vi "G#Object_Clone.vi"(0 "reference in":refnum<class "G#Object.lvclass">, 1 "new object name":string, 4 "no registration? (F)":bool, 5 "error in (no error)":errorcluster, 7 "user counter (T)?":bool=TRUE) -> (14 "reference out":refnum<class "G#Object.lvclass">, 16 "new object reference out":refnum<class "G#Object.lvclass">, 19 "error out":errorcluster)   [LabVIEW 2020, in "G#Object.lvclass"]
doc: "Clones the object specified by reference in and creates a new object with the identical state."
uses:
  G#Object.lvclass
  G#Object_State.ctl
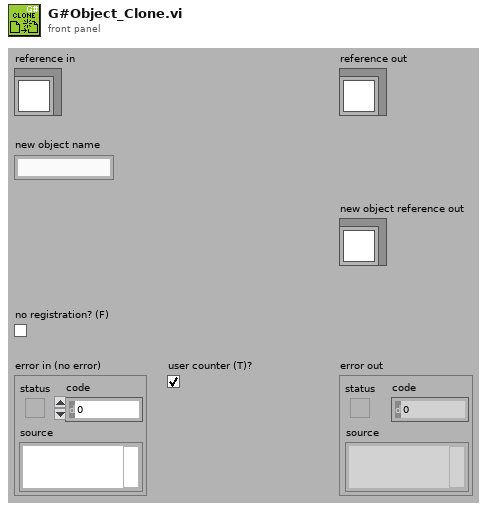
[diagram p1: front panel]
types:
  T1 = typedef "G#Object.lvclass/G#Object_State.ctl" = enum16{"Clear", "Create", "Delete", "Get class attributes", "Class hierarchy", "Get attribute value", "Set attribute value"}
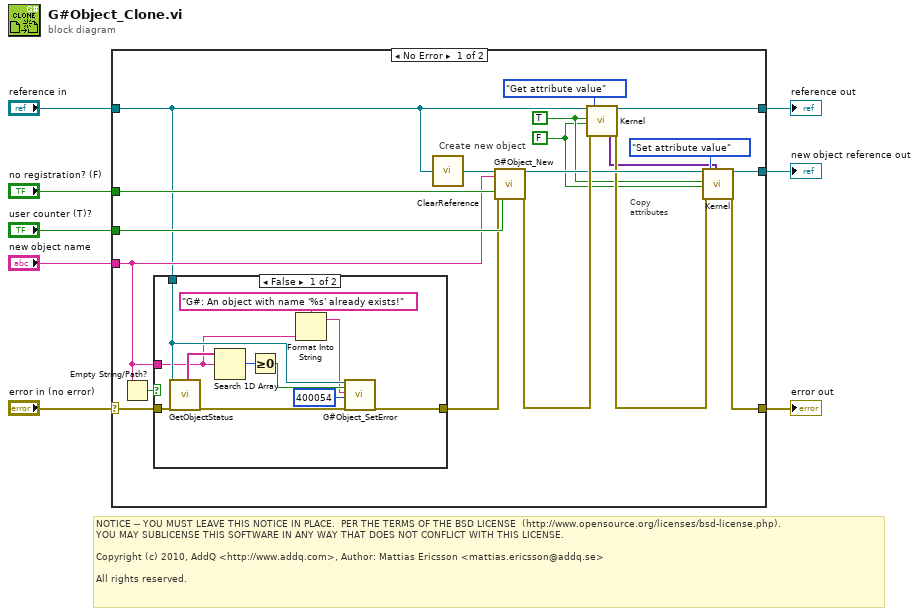
[diagram p0: block diagram]
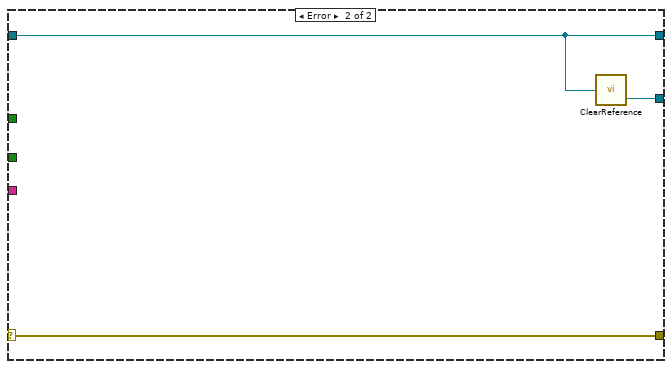
[diagram p3: hidden frame]
diagram:
  # "NOTICE -- YOU MUST LEAVE THIS NOTICE IN PLACE.  PER THE TERMS OF THE BSD LICENSE  (http://www.opensource.org/licenses/bsd-license.php).\nYOU MAY SUBLICENSE THIS SOFTWARE IN ANY WAY THAT DOES NOT CONFLICT WITH THIS LICENSE.\n\nCopyright (c) 2010, AddQ <http://www.addq.com>, Author: Mattias Ericsson <mattias.ericsson@addq.se>\n\nAll rights reserved."
  n1 = case shown="No Error" "error in (no error)" {
    selector: "error in (no error)" -> [w24 w42]
    tunnel: [w15 w42] -> w7
    tunnel: [w14 w40] -> w5
    tunnel: "reference in" -> [w20 w40]
    tunnel: "new object name" -> [w21 _]
    tunnel: "no registration? (F)" -> [w27 _]
    tunnel: "user counter (T)?" -> [w26 _]
    tunnel: [w18 w41] -> w1
    frame No Error {
      w9 = FALSE ("option 2")
      w10 = TRUE ("option 1")
      # "Copy\nattributes"
      # "Create new object"
      n2 = Empty String/Path?(string/path=w21) -> (empty?=w22:bool)
      n3 = case shown="False" w22 {
        tunnel: w24 -> [w38 w39]
        tunnel: [w35 w39] -> w23
        tunnel: w20 -> [w34 _]
        tunnel: w21 -> [w28 _]
        frame False {
          n4 = call-dynamic "GetObjectStatus.vi"("reference in"=w34, "error in (no error)"=w38) -> ("all object names"=w37:string[], "error out"=w36:errorcluster)  [unwired: 6 in, 10 out]
          n5 = Search 1D Array(1D array=w37, element=w28) -> (index of element=w33:i32)  [unwired: 1 in]
          n6 = Greater Or Equal To 0?(x=w33) -> (x >= 0?=w32:bool)
          n7 = Format Into String(format string="G#: An object with name '%s' already exists!", w28) -> (resulting string=w29:string)  [unwired: 2 in, 1 out]
          n8 = call "G#Object_SetError.vi"("reference in"=w34, "error (F)"=w32, "source"=w29, "code"=400054, "error in (no error)"=w36) -> ("error out"=w35:errorcluster)  [unwired: 14 in]
        }
        frame True {
        }
      }
      n9 = call-dynamic "ClearReference.vi"("reference in"=w20) -> ("reference out"=w25:refnum<class "G#Object.lvclass">)
      n10 = call "G#Object_New.vi"("reference in"=w25, "object name"=w21, "no registration? (F)"=w27, "error in (no error)"=w23, "user counter (T)?"=w26) -> ("reference out"=w17:refnum<class "G#Object.lvclass">, "error out"=w19:errorcluster)  [unwired: 12 in, 1 out]
      n11 = call-dynamic "Kernel.vi"("reference in"=w20, "option 1"=w10, "option 2"=w9, "error in (no error)"=w19, "state"=G#Object_State."Get attribute value") -> ("attributes out"=w11:variant[], "reference out"=w14:refnum<class "G#Object.lvclass">, "error out"=w16:errorcluster)  [unwired: 6 in, 6 out]
      n12 = call-dynamic "Kernel.vi"("reference in"=w17, "option 1"=w10, "option 2"=w9, "error in (no error)"=w16, "state"=G#Object_State."Set attribute value", "attributes in"=w11) -> ("reference out"=w18:refnum<class "G#Object.lvclass">, "error out"=w15:errorcluster)  [unwired: 5 in, 7 out]
    }
    frame Error {
      n13 = call-dynamic "ClearReference.vi"("reference in"=w40) -> ("reference out"=w41:refnum<class "G#Object.lvclass">)
    }
  }
  "error out" <- w7
  "reference out" <- w5
  "new object reference out" <- w1
